vi "Convert Integr to CBOR Hex.vi"(8 "error in (no error)":errorcluster, 11 "Integer":i32) -> (0 "error out":errorcluster, 3 "CBOR Hex":string)   [LabVIEW 2020, in "CBOR.lvlib"]
doc: "Convert intger data into CBOR hex data."
uses:
  CBOR.lvlib
  Controls/Structure Options.ctl
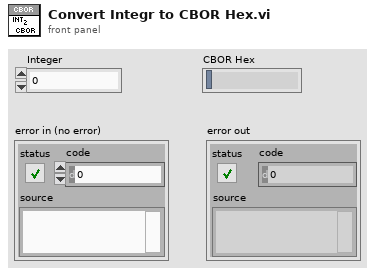
[diagram p1: front panel]
types:
  T1 = typedef "CBOR.lvlib/Structure Options.ctl" = enum16{"Map", "Text", "Array", "Integer", "Float"}
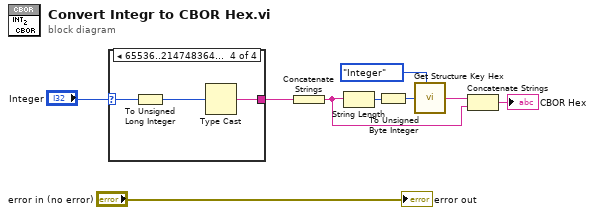
[diagram p0: block diagram]
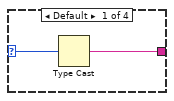
[diagram p2: hidden frame]
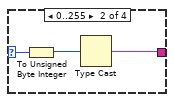
[diagram p3: hidden frame]
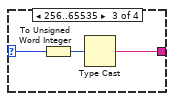
[diagram p4: hidden frame]
diagram:
  n1 = case shown="65536..2147483646" "Integer" {
    selector: "Integer" -> [w10 w14 w17 w20]
    tunnel: [w11 w13 w16 w19] -> w2
    frame Default {
      n2 = Type Cast(x=w10) -> (*(type *) &x=w11:string)  [unwired: 1 in]
    }
    frame 0..255 {
      n3 = To Unsigned Byte Integer(number=w14) -> (unsigned 8bit integer=w12:u8)
      n4 = Type Cast(x=w12) -> (*(type *) &x=w13:string)  [unwired: 1 in]
    }
    frame 256..65535 {
      n5 = To Unsigned Word Integer(number=w17) -> (unsigned 16bit integer=w15:u16)
      n6 = Type Cast(x=w15) -> (*(type *) &x=w16:string)  [unwired: 1 in]
    }
    frame 65536..2147483646 {
      n7 = To Unsigned Long Integer(number=w20) -> (unsigned 32bit integer=w18:u32)
      n8 = Type Cast(x=w18) -> (*(type *) &x=w19:string)  [unwired: 1 in]
    }
  }
  n9 = Concatenate Strings(w2) -> (w7:string)
  n10 = String Length(string=w7) -> (length=w1:i32)
  n11 = To Unsigned Byte Integer(number=w1) -> (unsigned 8bit integer=w4:u8)
  n12 = call "Get Structure Key Hex.vi"("Struct Options"=Structure_Options."Integer", "# Struct Elements"=w4) -> ("Key"=w8:string)  [unwired: 7 in]
  n13 = Concatenate Strings(w8, w7) -> (→"CBOR Hex":string)
  "error out" <- "error in (no error)"
